vi "completed_tracks_functional_gloabl.vi"(8 "error in (no error)":errorcluster, 10 "?":T3, 11 "CompletedTracksToSave":T1[](array[typedef])) -> (0 "error out":errorcluster, 1 "CompletedTrackCount":i32, 2 "LastTrackIndex":i32, 3 "OutputTracks":T1[](array[typedef]))   [LabVIEW 2019]
uses:
  CompletedTracksFunctionalGlobalOperations.ctl
  WormTrackCluster.ctl
  StimulusObject.lvclass
  TrackTerminationReasonEnum.ctl
  StimulusObject.lvclass/StimulusObject.ctl
  ParametersGlobal.vi
  DebugGlobal.vi
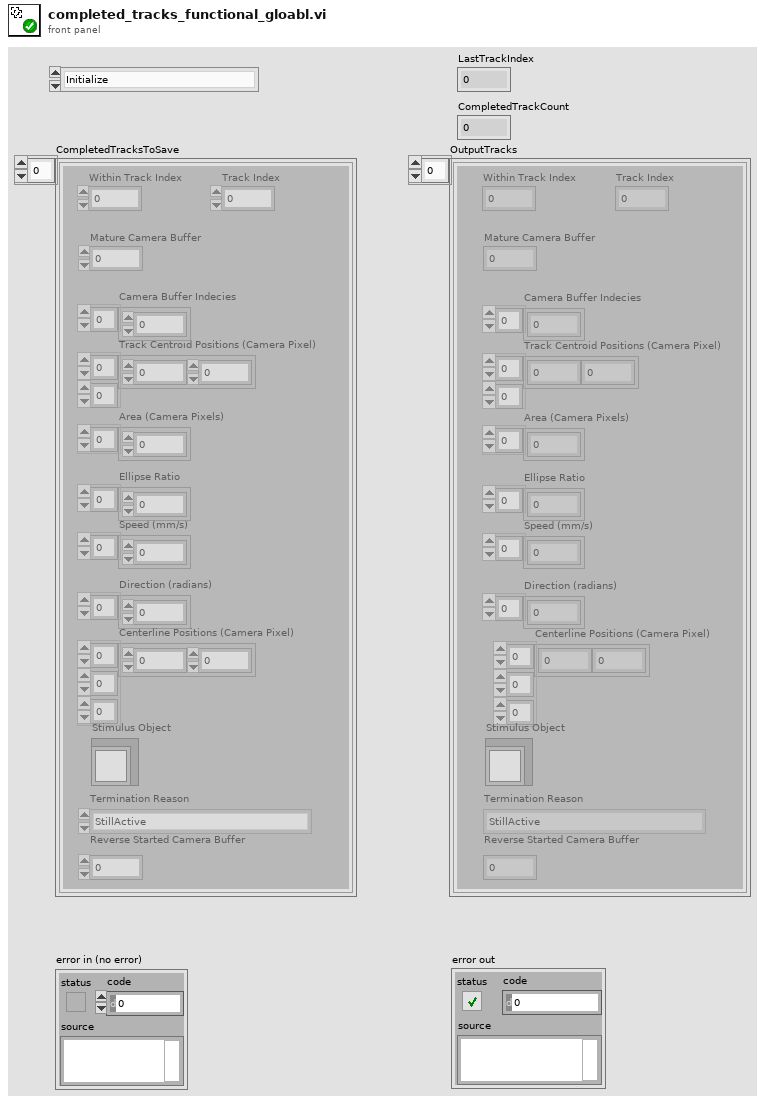
[diagram p1: front panel]
types:
  T1 = typedef "WormTrackCluster.ctl" = cluster{"Track Centroid Positions (Camera Pixel)":sgl[][], "Within Track Index":i32, "Camera Buffer Indecies":i32[], "Area (Camera Pixels)":i32[], "Speed (mm/s)":sgl[], "Direction (radians)":sgl[], "Centerline Positions (Camera Pixel)":sgl[][][], "Ellipse Ratio":sgl[], "Stimulus Object":refnum<class "StimulusObject.lvclass">, "Termination Reason":T2, "Track Index":i32, "Mature Camera Buffer":i32, "Reverse Started Camera Buffer":i32}
  T2 = typedef "TrackTerminationReasonEnum.ctl" = enum16{"StillActive", "MaxDisplacement", "NoBlobsLeft", "AreaIncrease", "AreaDecrease", "ExperimentEnded"}
  T3 = typedef "CompletedTracksFunctionalGlobalOperations.ctl" = enum16{"Initialize", "ReturnAllTracks", "ReturnLastIndex", "SaveCompletedTracks", "TrimAndReturnAllTracks"}
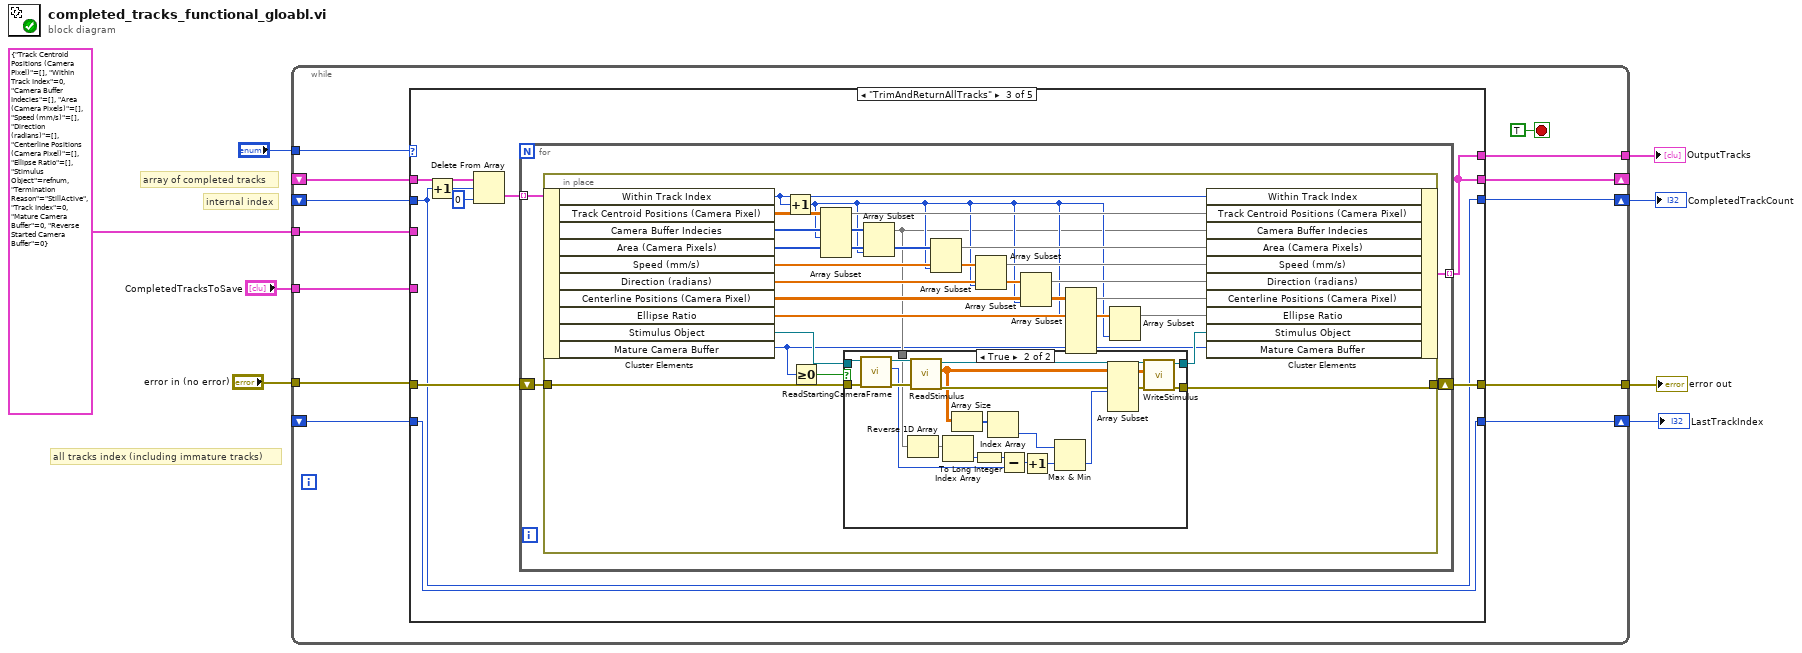
[diagram p0: block diagram]
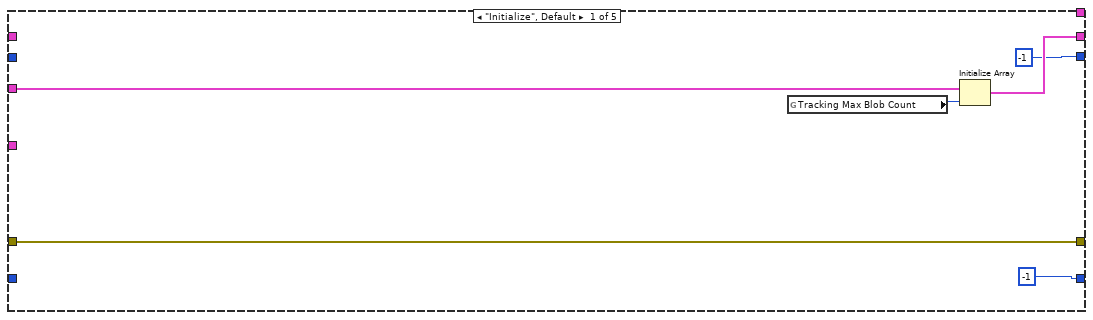
[diagram p2: hidden frame]
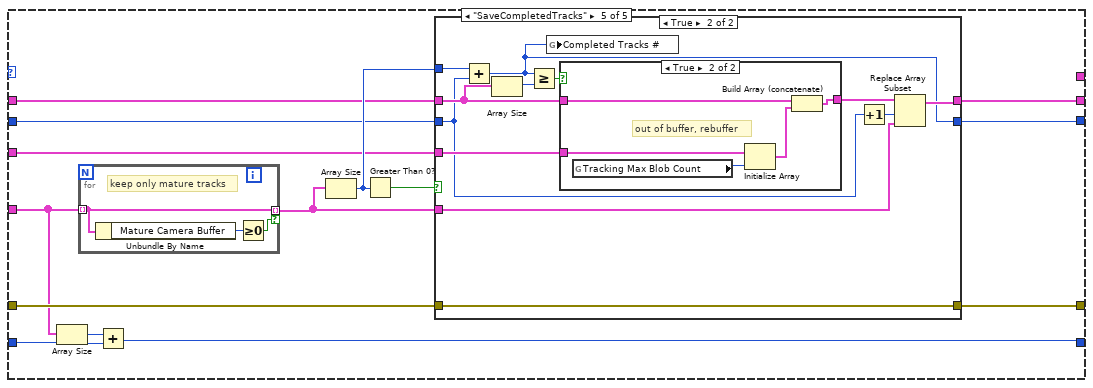
[diagram p6: hidden frame]
diagram:
  # "all tracks index (including immature tracks)"
  # "array of completed tracks"
  # "internal index"
  n1 = while {
    shift-right: [w11] -> w1
    shift-left: _ -> [w18]
    shift-right: [w17] -> _
    shift-left: _ -> [w19]
    tunnel: T1 {"Track Centroid Positions (Camera Pixel)"=[], "Within Track Index"=0, "Camera Buffer Indecies"=[], "Area (Camera Pixels)"=[], "Speed (mm/s)"=[], "Direction (radians)"=[], "Centerline Positions (Camera Pixel)"=[], "Ellipse Ratio"=[], "Stimulus Object"=refnum, "Termination Reason"=enum."StillActive", "Track Index"=0, "Mature Camera Buffer"=0, "Reverse Started Camera Buffer"=0} ("Tracks") -> [w20]
    tunnel: "?" -> [w16]
    tunnel: "error in (no error)" -> [w15]
    tunnel: "CompletedTracksToSave" -> [w14]
    tunnel: [w13] -> w4
    tunnel: [w12] -> w3
    shift-right: [w10] -> w2
    shift-left: _ -> [w9]
    stop <- TRUE stop-if-true
    n2 = case shown="\"TrimAndReturnAllTracks\"" w16 {
      tunnel: [-1 w29 w34 w92 w100] -> w11
      tunnel: w20 -> [w26 _ _ _ w102]
      tunnel: [w25 w30 w33 w90 w101] -> w17
      tunnel: w19 -> [_ w30 w40 w90 w104]
      tunnel: w18 -> [_ w29 w34 w92 w103]
      tunnel: w15 -> [w23 w31 w36 w91 w98]
      tunnel: [w23 w31 w35 w91 w99] -> w12
      tunnel: [_ w30 w33 _ _] -> w13
      tunnel: w14 -> [_ _ _ _ w96]
      tunnel: [-1 w28 w32 w89 w93] -> w10
      tunnel: w9 -> [_ w28 w32 w89 w94]
      frame "Initialize", Default {
        n3 = global read "ParametersGlobal.vi" "Tracking Max Blob Count"() -> (w27:i32)
        n4 = Initialize Array(w26, w27) -> (w25:T1[])
      }
      frame "ReturnAllTracks" {
      }
      frame "TrimAndReturnAllTracks" {
        n5 = Increment(x=w34) -> (x+1=w38:i32)
        n6 = Delete From Array(array=w40, length=w38, index=0) -> (deleted portion=w37:T1[])  [unwired: 1 out]
        n7 = for {
          tunnel: w37 -> [w44] mode=indexing
          tunnel: [w43] -> w33 mode=indexing
          shift-right: [w41] -> w35
          shift-left: w36 -> [w42]
          n8 = in-place {
            in-place-border: w42 -> [w51]
            in-place-border: [w50] -> w41
            n9 = in-place-cluster #1(w44) -> ("Within Track Index"=w65:i32, "Track Centroid Positions (Camera Pixel)"=w66:sgl[][], "Camera Buffer Indecies"=w63:i32[], "Area (Camera Pixels)"=w62:i32[], "Speed (mm/s)"=w61:sgl[], "Direction (radians)"=w60:sgl[], "Centerline Positions (Camera Pixel)"=w59:sgl[][][], "Ellipse Ratio"=w58:sgl[], "Stimulus Object"=w49:refnum<class "StimulusObject.lvclass">, "Mature Camera Buffer"=w45:i32)
            n10 = Increment(x=w65) -> (x+1=w53:i32)
            n11 = Greater Or Equal To 0?(x=w45) -> (x >= 0?=w46:bool)
            n12 = Array Subset(array=w66, length (row)=w53) -> (w64:sgl[][])  [unwired: 3 in]
            n13 = Array Subset(array=w63, length=w53) -> (w47:i32[])  [unwired: 1 in]
            n14 = case shown="True" w46 {
              tunnel: w51 -> [w68 w79]
              tunnel: [w68 w78] -> w50
              tunnel: w49 -> [w67 w77]
              tunnel: [w67 w76] -> w48
              tunnel: w47 -> [_ w75]
              frame False {
              }
              frame True {
                n15 = call "ReadStartingCameraFrame.vi"("error in (no error)"=w79, "StimulusObject in"=w77) -> ("error out"=w88:errorcluster, "StartingCameraFrame"=w80:i32, "StimulusObject out"=w87:refnum<class "StimulusObject.lvclass">)  [unwired: 7 in]
                n16 = Reverse 1D Array(array=w75) -> (reversed array=w86:i32[])
                n17 = call "ReadStimulus.vi"("error in (no error)"=w88, "StimulusObject in"=w87) -> ("error out"=w82:errorcluster, "StimulusOut"=w74:sgl[][], "StimulusObject out"=w85:refnum<class "StimulusObject.lvclass">)  [unwired: 7 in]
                n18 = Index Array(array=w86) -> (element=w81:i32)  [unwired: 1 in]
                n19 = Array Size(array=w74) -> (size(s)=w72:i32[])
                n20 = To Long Integer(number=w81) -> (32bit integer=w73:i32)
                n21 = Index Array(array=w72) -> (element=w71:i32)  [unwired: 1 in]
                n22 = Subtract(x=w73, y=w80) -> (x-y=w84:i32)
                n23 = Increment(x=w84) -> (x+1=w70:i32)
                n24 = Max & Min(x=w71, y=w70) -> (min(x,y)=w69:i32)  [unwired: 1 out]
                n25 = Array Subset(array=w74, length (row)=w69) -> (w83:sgl[][])  [unwired: 3 in]
                n26 = call "WriteStimulus.vi"("error in (no error)"=w82, "Stimulus"=w83, "StimulusObject in"=w85) -> ("error out"=w78:errorcluster, "StimulusObject out"=w76:refnum<class "StimulusObject.lvclass">)  [unwired: 7 in]
              }
            }
            n27 = Array Subset(array=w62, length=w53) -> (w57:i32[])  [unwired: 1 in]
            n28 = Array Subset(array=w61, length=w53) -> (w56:sgl[])  [unwired: 1 in]
            n29 = Array Subset(array=w60, length=w53) -> (w55:sgl[])  [unwired: 1 in]
            n30 = Array Subset(array=w59, length (dim 0)=w53) -> (w54:sgl[][][])  [unwired: 5 in]
            n31 = Array Subset(array=w58, length=w53) -> (w52:sgl[])  [unwired: 1 in]
            n32 = in-place-cluster #1("Within Track Index"=w65, "Track Centroid Positions (Camera Pixel)"=w64, "Camera Buffer Indecies"=w47, "Area (Camera Pixels)"=w57, "Speed (mm/s)"=w56, "Direction (radians)"=w55, "Centerline Positions (Camera Pixel)"=w54, "Ellipse Ratio"=w52, "Stimulus Object"=w48, "Mature Camera Buffer"=w45) -> (w43:T1)
          }
        }
      }
      frame "ReturnLastIndex" {
      }
      frame "SaveCompletedTracks" {
        n33 = Array Size(array=w96) -> (size(s)=w95:i32)
        n34 = for {
          tunnel: w96 -> [w108] mode=indexing
          tunnel: [w108] -> w97 mode=indexing if=w107
          # "keep only mature tracks"
          n35 = Unbundle By Name(w108) -> ("Mature Camera Buffer"=w109:i32)
          n36 = Greater Or Equal To 0?(x=w109) -> (x >= 0?=w107:bool)
        }
        n37 = Add(x=w95, y=w94) -> (x+y=w93:i32)
        n38 = Array Size(array=w97) -> (size(s)=w105:i32)
        n39 = Greater Than 0?(x=w105) -> (x > 0?=w106:bool)
        n40 = case shown="True" w106 {
          tunnel: w97 -> [_ w116]
          tunnel: w105 -> [_ w124]
          tunnel: w104 -> [w112 w121]
          tunnel: w103 -> [w111 w117]
          tunnel: w102 -> [_ w120]
          tunnel: [w112 w115] -> w101
          tunnel: [w111 w113] -> w100
          tunnel: [w110 w114] -> w99
          tunnel: w98 -> [w110 w114]
          frame False {
          }
          frame True {
            n41 = Add(x=w124, y=w117) -> (x+y=w113:i32)
            n42 = Array Size(array=w121) -> (size(s)=w123:i32)
            n43 = Greater Or Equal?(x=w113, y=w123) -> (x >= y?=w122:bool)
            n44 = global write "DebugGlobal.vi" "Completed Tracks #"(w113) -> ()
            n45 = case shown="True" w122 {
              tunnel: w121 -> [w125 w130]
              tunnel: w120 -> [_ w128]
              tunnel: [w125 w126] -> w119
              frame False {
              }
              frame True {
                # "out of buffer, rebuffer"
                n46 = global read "ParametersGlobal.vi" "Tracking Max Blob Count"() -> (w129:i32)
                n47 = Initialize Array(w128, w129) -> (w127:T1[])
                n48 = Build Array (concatenate)(w130, w127) -> (w126:T1[])
              }
            }
            n49 = Increment(x=w117) -> (x+1=w118:i32)
            n50 = Replace Array Subset(array=w119, new element=w116, index=w118) -> (w115:T1[])
          }
        }
      }
    }
  }
  "OutputTracks" <- w4
  "error out" <- w3
  "LastTrackIndex" <- w2
  "CompletedTrackCount" <- w1
